vi "Set Frequency.vi"(8 "error in (no error)":errorcluster, 11 "Harmonics in":refnum<class "Harmonics.lvclass">) -> (0 "error out":errorcluster, 1 "Parameter":cluster{"Name":string, "Value":string}, 2 "Last Frequency?":bool, 3 "Harmonics out":refnum<class "Harmonics.lvclass">)   [LabVIEW 2020, in "Harmonics.lvclass"]
uses:
  Harmonics.lvclass
  Harmonics.lvclass/Harmonics.ctl
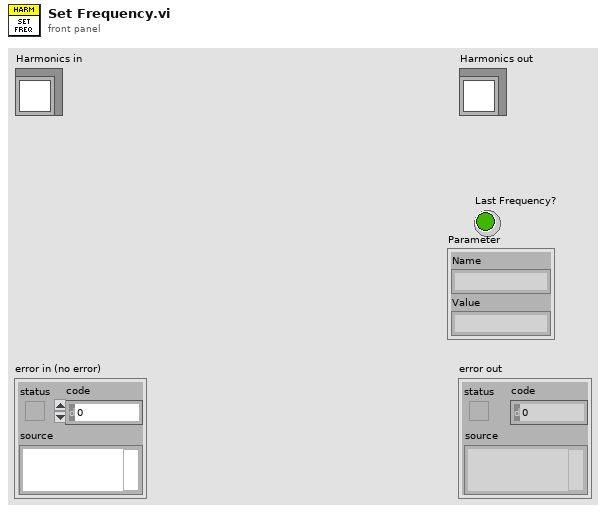
[diagram p1: front panel]
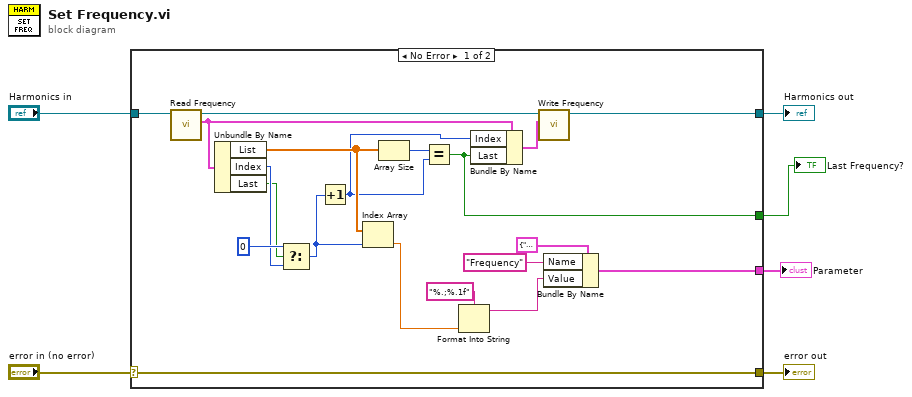
[diagram p0: block diagram]
diagram:
  n1 = case shown="No Error" "error in (no error)" {
    selector: "error in (no error)" -> [w7 w28]
    tunnel: [w7 w28] -> w5
    tunnel: [w8 w27] -> w3
    tunnel: "Harmonics in" -> [w26 w27]
    tunnel: [w15 _] -> w2
    tunnel: [w9 _] -> w1
    frame No Error {
      n2 = call "Read Frequency.vi"("Harmonics in"=w26) -> ("Frequency"=w24:cluster{"List":dbl[], "Index":i32, "Last":bool}, "Harmonics out"=w25:refnum<class "Harmonics.lvclass">)  [unwired: 9 in]
      n3 = Unbundle By Name(w24) -> ("List"=w19:dbl[], "Index"=w22:i32, "Last"=w20:bool)
      n4 = Select(t=0, s=w20, f=w22) -> (s? t:f=w17:i32)
      n5 = Increment(x=w17) -> (x+1=w16:i32)
      n6 = Index Array(array=w19, index=w17) -> (element=w10:dbl)
      n7 = Array Size(array=w19) -> (size(s)=w18:i32)
      n8 = Equal?(x=w18, y=w16) -> (x = y?=w15:bool)
      n9 = Format Into String(format string="%.;%.1f", w10) -> (resulting string=w11:string)  [unwired: 2 in, 1 out]
      n10 = Bundle By Name(cluster=w24, "Index"=w16, "Last"=w15) -> (w21:cluster{"List":dbl[], "Index":i32, "Last":bool})
      n11 = call "Write Frequency.vi"("Frequency"=w21, "Harmonics in"=w25) -> ("Harmonics out"=w8:refnum<class "Harmonics.lvclass">)  [unwired: 9 in]
      n12 = Bundle By Name(cluster=cluster{"Name":string, "Value":string} {"Name"="", "Value"=""} ("Change"), "Name"="Frequency", "Value"=w11) -> (w9:cluster{"Name":string, "Value":string})
    }
    frame Error {
    }
  }
  "error out" <- w5
  "Harmonics out" <- w3
  "Last Frequency?" <- w2
  "Parameter" <- w1
